vi "API_StageMoveToLoadPosition.vi"(6 "Timeout (ms)":u32=600000, 7 "Wait (F)":bool, 8 "error in (no error)":errorcluster, 9 "Task ID":string, 11 "Motor Controller in":refnum<class "Motor Controller.lvclass">) -> (0 "error out":errorcluster, 2 "Return Value":variant, 3 "Motor Controller out":refnum<class "Motor Controller.lvclass">)   [LabVIEW 2022 SP3, in "Motor Controller.lvclass"]
uses:
  Motor Controller.lvclass
  Typedefs/API Command Cluster.ctl
  Typedefs/API Command Enum.ctl
  Typedefs/SetExplicitMessage API Data.ctl
  Typedefs/Motor Controller Parameter-Set.ctl
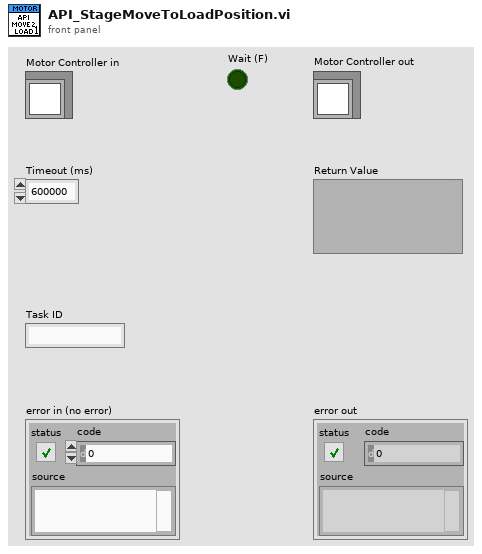
[diagram p1: front panel]
types:
  T1 = typedef "Motor Controller.lvclass/SetExplicitMessage API Data.ctl" = cluster{"Motor Controller Parameter":T2, "value":i32}
  T2 = typedef "Motor Controller.lvclass/Motor Controller Parameter-Set.ctl" = enum16{"Print Speed", "Jog Speed", "PR Path", "Enable Servo", "Disable Servo", "Move Stage to Under PH1", "Move Stage to Under PH2", "Move Stage to Under PH3", "Move Stage to Under PH4", "Move Stage to Under PH5", "Move Stage to Under PH6", "Home Stage", "Return Stage to 0", "Print Stage", "Write Speed", "Write Index", "Stop Stage"}
  T3 = typedef "Motor Controller.lvclass/API Command Enum.ctl" = enum16{"GetExplicitMessage", "SetExplicitMessage", "Execute Stage Move Recipe", "Read Stage Move Recipe", "Abort"}
  T4 = typedef "Motor Controller.lvclass/API Command Cluster.ctl" = cluster{"Command":T3, "Arguments":string, "Data":variant}
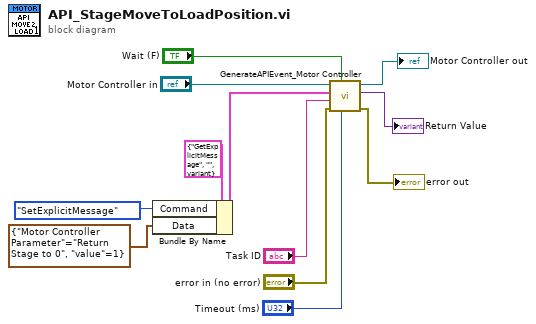
[diagram p0: block diagram]
diagram:
  n1 = Bundle By Name(cluster=T4 {"Command"=enum."GetExplicitMessage", "Arguments"="", "Data"=variant} ("API Command Cluster"), "Command"=API_Command_Enum."SetExplicitMessage", "Data"=T1 {"Motor Controller Parameter"=enum."Return Stage to 0", "value"=1} ("SetExplicitMessage API Data")) -> (w4:T4)
  n2 = call-dynamic "GenerateAPIEvent_Motor Controller.vi"("Timeout (ms)"="Timeout (ms)", "Wait (F)"="Wait (F)", "error in (no error)"="error in (no error)", "Task ID"="Task ID", "API Command Cluster"=w4, "Motor Controller In"="Motor Controller in") -> ("error out"=→"error out":errorcluster, "Return Value"=→"Return Value":variant, "Motor Controller out"=→"Motor Controller out":refnum<class "Motor Controller.lvclass">)  [unwired: 3 in]
